vi "Add Log File.vi"(8 "error in":errorcluster, 10 "log file name":string="Log File", 11 "embedded data logger in":T1=18446744073709551615 format="%.0x") -> (0 "error out":errorcluster, 2 "log file":T1 format="%.0x", 3 "embedded data logger out":T1 format="%.0x")   [LabVIEW 2027, in "Embedded Data Logger Scripting.lvlib"]
uses:
  Embedded Data Logger Scripting.lvlib
  <vilib>/NI VeriStand/Custom Device API/Custom Device Item Ref.ctl
  <vilib>/NI VeriStand/Custom Device API/Custom Device Channel.ctl
  <vilib>/NI VeriStand/Custom Device API/Custom Device Channel Type.ctl
  Shared/Constants.vi
  <vilib>/NI VeriStand/Custom Device API/Custom Device API.lvlib
  Shared/Embedded Data Logger Shared.lvlib
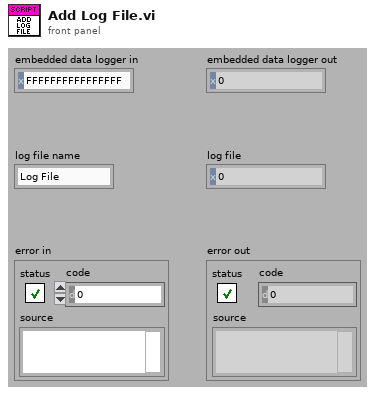
[diagram p1: front panel]
types:
  T1 = typedef "Custom Device API.lvlib/Custom Device Item Ref.ctl" = u64
  T2 = typedef "Custom Device API.lvlib/Custom Device Channel Type.ctl" = enum16{"Input", "Output"}
  T3 = typedef "Custom Device API.lvlib/Custom Device Channel.ctl" = cluster{"Type":T2, "Units":string, "Default Value":dbl, "Faultable":bool, "Scalable":bool}
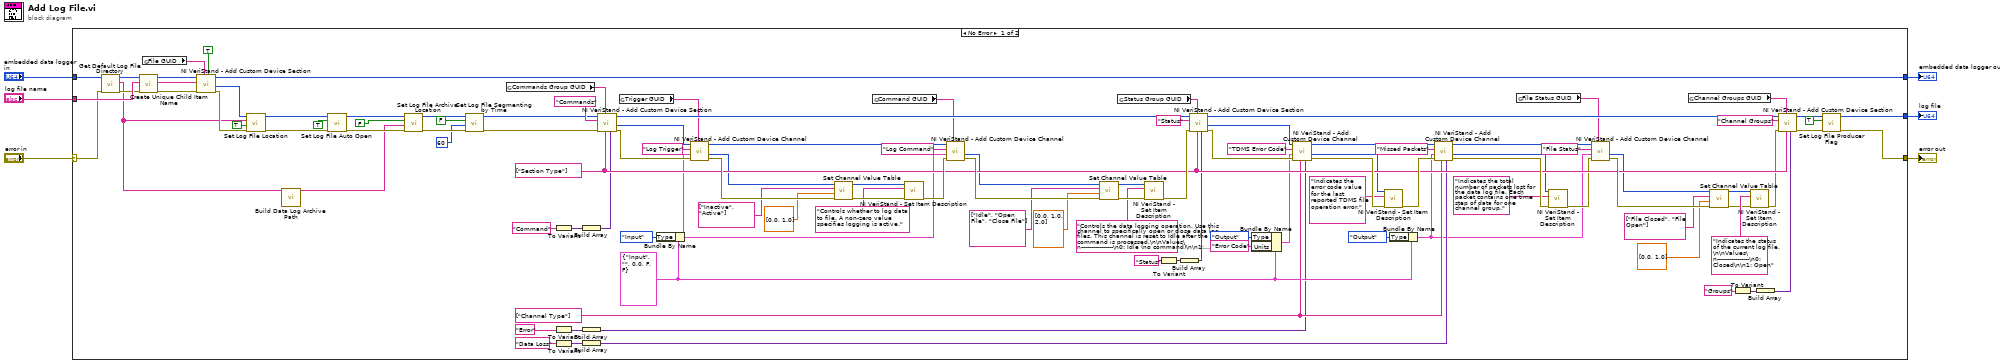
[diagram p0: block diagram]
diagram:
  n1 = case shown="No Error" "error in" {
    selector: "error in" -> [w78 w120]
    tunnel: "log file name" -> [w103 _]
    tunnel: "embedded data logger in" -> [w15 w121]
    tunnel: [w12 w121] -> w4
    tunnel: [w8 w120] -> w3
    tunnel: [w7 _] -> w1
    frame No Error {
      w105 = string[] ["Channel Type"] ("Property names")
      w72 = T3 {"Type"=enum."Input", "Units"="", "Default Value"=0.0, "Faultable"=FALSE, "Scalable"=FALSE} ("Channel")
      w106 = string[] ["Section Type"] ("Property names")
      n2 = call "Get Default Log File Directory.vi"("error in"=w78, "Device Item Ref In"=w15) -> ("error out"=w16:errorcluster, "Log File Directory String Array"=w13:string[], "Device Item Ref Out"=w14:T1)  [unwired: 7 in]
      n3 = call "Create Unique Child Item Name.vi"("error in (no error)"=w16, "Name in"=w103, "Parent Item Ref in"=w14) -> ("error out"=w102:errorcluster, "Unique Name out"=w100:string, "Parent Item Ref out"=w101:T1)  [unwired: 6 out]
      n4 = global read "Constants.vi" "File GUID"() -> (w31:string)
      n5 = call <vilib>:"NI VeriStand - Add Custom Device Section.vi"("Highlight? (F)"=TRUE, "GUID (Default Section)"=w31, "error in (no error)"=w102, "Section Name"=w100, "Parent Ref in"=w101) -> ("error out"=w104:errorcluster, "Section Ptr"=w98:T1, "Parent Ref out"=w12:T1)  [unwired: 2 in, 2 out]
      n6 = call "Set Log File Location.vi"("error in"=w104, "timestamp file name"=TRUE, "directory parts"=w13, "log file in"=w98) -> ("error out"=w52:errorcluster, "log file out"=w53:T1)  [unwired: 5 in, 1 out]
      n7 = call "Build Data Log Archive Path.vi"("Log Directory String Array"=w13) -> ("Log Archive Directory String Array"=w23:string[])  [unwired: 14 in]
      n8 = call "Set Log File Auto Open.vi"("error in"=w52, "auto open"=TRUE ("Value"), "log file in"=w53) -> ("error out"=w26:errorcluster, "log file out"=w24:T1)  [unwired: 7 in]
      n9 = call "Set Log File Archive Location.vi"("error in (no error)"=w26, "archive directory parts"=w23, "archive closed log files"=FALSE ("Value"), "log file in"=w24) -> ("error out"=w22:errorcluster, "log file out"=w21:T1)  [unwired: 6 in]
      n10 = call "Set Log File Segmenting by Time.vi"("error in"=w22, "file length (s)"=u32 60 ("Default Value"), "segment into multiple files"=FALSE ("Value"), "log file in"=w21) -> ("error out"=w20:errorcluster, "log file out"=w19:T1)  [unwired: 6 in]
      n11 = global read "Constants.vi" "Commands Group GUID"() -> (w17:string)
      n12 = To Variant(anything="Command" ("String")) -> (Variant=w96:variant)
      n13 = To Variant(anything="Error" ("String")) -> (Variant=w76:variant)
      n14 = To Variant(anything="Data Loss" ("String")) -> (Variant=w71:variant)
      n15 = Build Array(w96) -> (w97:variant[])
      n16 = Build Array(w76) -> (w68:variant[])
      n17 = Build Array(w71) -> (w69:variant[])
      n18 = call <vilib>:"NI VeriStand - Add Custom Device Section.vi"("Property Values"=w97, "Property names"=w106, "GUID (Default Section)"=w17, "error in (no error)"=w20, "Section Name"="Commands", "Parent Ref in"=w19) -> ("error out"=w93:errorcluster, "Section Ptr"=w94:T1, "Parent Ref out"=w89:T1)  [unwired: 1 in, 2 out]
      n19 = global read "Constants.vi" "Trigger GUID"() -> (w30:string)
      n20 = Bundle By Name(cluster=w72, "Type"=Custom_Device_Channel_Type."Input") -> (w55:T3)
      n21 = call <vilib>:"NI VeriStand - Add Custom Device Channel.vi"("GUID (Default Channel)"=w30, "error in (no error)"=w93, "Channel"=w55, "Channel Name"="Log Trigger", "Parent Ref in"=w94) -> ("error out"=w117:errorcluster, "Channel Ref"=w37:T1, "Parent Ref out"=w56:T1)  [unwired: 3 in, 1 out]
      n22 = call "Set Channel Value Table.vi"("error in"=w117, "values"=dbl[] [0.0, 1.0] ("Values"), "names"=string[] ["Inactive", "Active"] ("Names"), "channel in"=w37) -> ("error out"=w113:errorcluster, "channel out"=w38:T1)  [unwired: 6 in]
      n23 = global read "Constants.vi" "Command GUID"() -> (w29:string)
      n24 = call <vilib>:"NI VeriStand - Set Item Description.vi"("error in (no error)"=w113, "Description"="Controls whether to log data to file. A non-zero value specifies logging is active." ("String"), "Item Ref in"=w38) -> ("error out"=w111:errorcluster)  [unwired: 6 in, 2 out]
      n25 = call <vilib>:"NI VeriStand - Add Custom Device Channel.vi"("GUID (Default Channel)"=w29, "error in (no error)"=w111, "Channel"=w55, "Channel Name"="Log Command", "Parent Ref in"=w56) -> ("error out"=w118:errorcluster, "Channel Ref"=w41:T1)  [unwired: 3 in, 2 out]
      n26 = call "Set Channel Value Table.vi"("error in"=w118, "values"=dbl[] [0.0, 1.0, 2.0] ("Values"), "names"=string[] ["Idle", "Open File", "Close File"] ("Names"), "channel in"=w41) -> ("error out"=w112:errorcluster, "channel out"=w40:T1)  [unwired: 6 in]
      n27 = global read "Constants.vi" "Status Group GUID"() -> (w18:string)
      n28 = call <vilib>:"NI VeriStand - Set Item Description.vi"("error in (no error)"=w112, "Description"="Controls the data logging operation. Use this channel to specifically open or close data log files. This channel is reset to Idle after the command is processed.\n\nValues\n----------------\n0: Idle (no command)\n\n1: Open File. Closes the previous file reference if it was open and opens a new file reference.\n\n2: Close File. Closes the file reference without opening a new file reference." ("String"), "Item Ref in"=w40) -> ("error out"=w110:errorcluster)  [unwired: 6 in, 2 out]
      n29 = To Variant(anything="Status" ("String")) -> (Variant=w88:variant)
      n30 = Build Array(w88) -> (w87:variant[])
      n31 = call <vilib>:"NI VeriStand - Add Custom Device Section.vi"("Property Values"=w87, "Property names"=w106, "GUID (Default Section)"=w18, "error in (no error)"=w110, "Section Name"="Status", "Parent Ref in"=w89) -> ("error out"=w84:errorcluster, "Section Ptr"=w85:T1, "Parent Ref out"=w67:T1)  [unwired: 1 in, 2 out]
      n32 = Bundle By Name(cluster=w72, "Type"=Custom_Device_Channel_Type."Output", "Units"="Error Code") -> (w81:T3)
      n33 = call <vilib>:"NI VeriStand - Add Custom Device Channel.vi"("Property Values"=w68, "Property names"=w105, "error in (no error)"=w84, "Channel"=w81, "Channel Name"="TDMS Error Code", "Parent Ref in"=w85) -> ("error out"=w109:errorcluster, "Channel Ref"=w61:T1, "Parent Ref out"=w75:T1)  [unwired: 2 in, 1 out]
      n34 = call <vilib>:"NI VeriStand - Set Item Description.vi"("error in (no error)"=w109, "Description"="Indicates the error code value for the last reported TDMS file operation error." ("String"), "Item Ref in"=w61) -> ("error out"=w107:errorcluster)  [unwired: 6 in, 2 out]
      n35 = Bundle By Name(cluster=w72, "Type"=Custom_Device_Channel_Type."Output") -> (w47:T3)
      n36 = call <vilib>:"NI VeriStand - Add Custom Device Channel.vi"("Property Values"=w69, "Property names"=w105, "error in (no error)"=w107, "Channel"=w47, "Channel Name"="Missed Packets", "Parent Ref in"=w75) -> ("error out"=w108:errorcluster, "Channel Ref"=w59:T1, "Parent Ref out"=w49:T1)  [unwired: 2 in, 1 out]
      n37 = global read "Constants.vi" "File Status GUID"() -> (w28:string)
      n38 = call <vilib>:"NI VeriStand - Set Item Description.vi"("error in (no error)"=w108, "Description"="Indicates the total number of packets lost for the data log file. Each packet contains one time step of data for one channel group." ("String"), "Item Ref in"=w59) -> ("error out"=w48:errorcluster)  [unwired: 6 in, 2 out]
      n39 = call <vilib>:"NI VeriStand - Add Custom Device Channel.vi"("GUID (Default Channel)"=w28, "error in (no error)"=w48, "Channel"=w47, "Channel Name"="File Status", "Parent Ref in"=w49) -> ("error out"=w119:errorcluster, "Channel Ref"=w33:T1)  [unwired: 3 in, 2 out]
      n40 = global read "Constants.vi" "Channel Groups GUID"() -> (w27:string)
      n41 = call "Set Channel Value Table.vi"("error in"=w119, "values"=dbl[] [0.0, 1.0] ("Values"), "names"=string[] ["File Closed", "File Open"] ("Names"), "channel in"=w33) -> ("error out"=w35:errorcluster, "channel out"=w34:T1)  [unwired: 6 in]
      n42 = To Variant(anything="Groups" ("String")) -> (Variant=w64:variant)
      n43 = call <vilib>:"NI VeriStand - Set Item Description.vi"("error in (no error)"=w35, "Description"="Indicates the status of the current log file.\n\nValues\n----------------\n0: Closed\n\n1: Open" ("String"), "Item Ref in"=w34) -> ("error out"=w45:errorcluster)  [unwired: 6 in, 2 out]
      n44 = Build Array(w64) -> (w63:variant[])
      n45 = call <vilib>:"NI VeriStand - Add Custom Device Section.vi"("Property Values"=w63, "Property names"=w106, "GUID (Default Section)"=w27, "error in (no error)"=w45, "Section Name"="Channel Groups", "Parent Ref in"=w67) -> ("error out"=w43:errorcluster, "Parent Ref out"=w44:T1)  [unwired: 1 in, 3 out]
      n46 = call "Set Log File Producer Flag.vi"("error in"=w43, "log file producer"=TRUE ("Log File Provider"), "custom device item in"=w44) -> ("error out"=w8:errorcluster, "custom device item out"=w7:T1)  [unwired: 7 in]
    }
    frame Error {
    }
  }
  "embedded data logger out" <- w4
  "error out" <- w3
  "log file" <- w1
